vi "Simple Resizing.vi"() -> ()   [LabVIEW 2012]
uses:
  vi.lib/Front Panel Layout/Scaling Settings.ctl
  vi.lib/Front Panel Layout/Scaling Type.ctl
  vi.lib/Front Panel Layout/VI Panel Layout/VI Panel Layout.lvclass
  vi.lib/Front Panel Layout/NI_SE_Front Panel Layout.lvlib
panel:
  in  "Scale Text":bool
  in  "OK Button":bool
  in  "Cluster":cluster{"String":string, "OK Button":bool}
  in  "Numeric":dbl
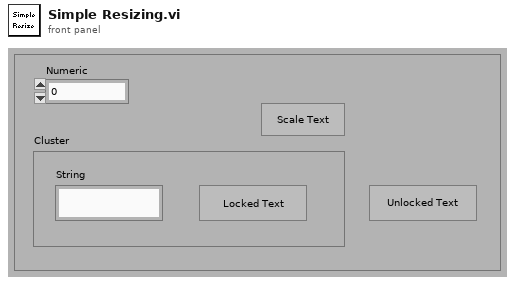
[diagram p1: front panel]
types:
  T1 = typedef "NI_SE_Front Panel Layout.lvlib/Scaling Settings.ctl" = cluster{"scaling type":T2, "scale text":bool}
  T2 = typedef "NI_SE_Front Panel Layout.lvlib/Scaling Type.ctl" = enum16{"None", "Scale panel to fit layout", "Scale layout to fit panel"}
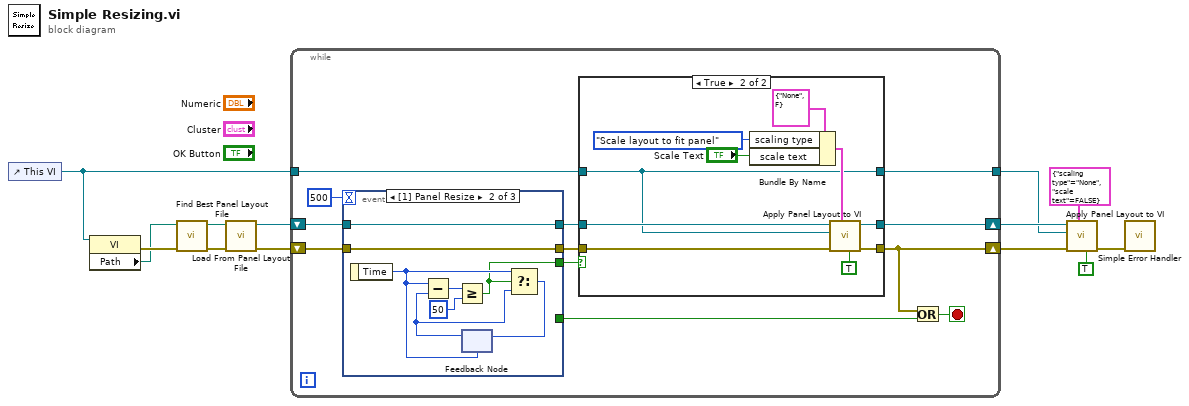
[diagram p0: block diagram]
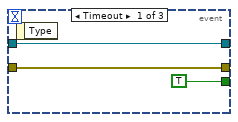
[diagram p3: hidden frame]
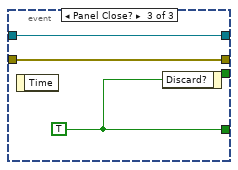
[diagram p4: hidden frame]
diagram:
  n1 = control-ref of="This VI"() -> (w7:refnum<vi>)
  n2 = property class="VI"(reference=w7) -> (error out=w11:errorcluster, "Path"=w10:path)  [unwired: 1 in, 1 out]
  n3 = call "Find Best Panel Layout File.vi"("error in"=w11, "VI path"=w10) -> ("error out"=w13:errorcluster, "panel layout file"=w12:path)  [unwired: 7 in, 1 out]
  n4 = call "Load From Panel Layout File.vi"("error in"=w13, "panel layout file"=w12) -> ("error out"=w9:errorcluster, "panel layout out"=w8:refnum<class "VI Panel Layout.lvclass">)  [unwired: 8 in]
  n5 = while {
    shift-right: [w14] -> w3
    shift-left: w9 -> [w23]
    tunnel: w7 -> [w16]
    shift-right: [w18] -> w4
    shift-left: w8 -> [w24]
    tunnel: [w15] -> w1
    stop <- w22 stop-if-true
    n6 = event shown="[1] Panel Resize" {
      selector: _ -> [_ _ _]
      dyn-events: _ -> [_ _ _]
      timeout: 500 -> [_ _ _]
      tunnel: w24 -> [w40 w49 w51]
      tunnel: w23 -> [w41 w48 w50]
      tunnel: [w41 w48 w50] -> w20
      tunnel: [_ _ w52] -> w21
      tunnel: [w40 w49 w51] -> w19
      tunnel: [TRUE w42 _] -> w17
      event Timeout {
        n7 = event-data() -> ()  [unwired: 1 in, 1 out]
      }
      event Panel Resize {
        n8 = event-data() -> ("Time"=w44:u32)  [unwired: 1 in]
        n9 = feedback #1(w44) -> (w45:u32)
        n10 = Subtract(x=w44, y=w45) -> (x-y=w47:u32)
        n11 = Greater Or Equal?(x=w47, y=u32 50) -> (x >= y?=w42:bool)
        n12 = Select(t=w44, s=w42, f=w45) -> (s? t:f=w43:u32)
        n13 = feedback-in #1(w43) -> ()
      }
      event Panel Close? {
        w52 = TRUE ("Discard?")
        n14 = event-data() -> ()  [unwired: 1 in, 1 out]
        n15 = event-data("Discard?"=w52) -> ()  [unwired: 1 in, 1 out]
      }
    }
    n16 = case shown="True" w17 {
      tunnel: w19 -> [w27 w38]
      tunnel: w20 -> [w28 w37]
      tunnel: [w28 w35] -> w14
      tunnel: [w27 w34] -> w18
      tunnel: w16 -> [w26 w29]
      tunnel: [w26 w29] -> w15
      frame False {
      }
      frame True {
        n17 = Bundle By Name(cluster=T1 {"scaling type"=enum."None", "scale text"=FALSE} ("scaling settings"), "scaling type"=Scaling_Type."Scale layout to fit panel", "scale text"="Scale Text") -> (w31:T1)
        n18 = call "Apply Panel Layout to VI.vi"("defer panel updates (F)"=TRUE, "scaling settings"=w31, "error in"=w37, "VI refnum"=w29, "panel layout in"=w38) -> ("error out"=w35:errorcluster, "panel layout out"=w34:refnum<class "VI Panel Layout.lvclass">)  [unwired: 5 in]
      }
    }
    n19 = Or(x=w14, y=w21) -> (x .or. y?=w22:bool)
  }
  n20 = call "Apply Panel Layout to VI.vi"("defer panel updates (F)"=TRUE, "scaling settings"=T1 {"scaling type"=enum."None", "scale text"=FALSE}, "error in"=w3, "VI refnum"=w1, "panel layout in"=w4) -> ("error out"=w2:errorcluster)  [unwired: 5 in, 1 out]
  n21 = call <vilib>:"Simple Error Handler.vi"("error in (no error)"=w2) -> ()  [unwired: 4 in, 5 out]
